vi "Write Averaging time.vi"(8 "error in (no error)":errorcluster, 10 "Time constant":dbl, 11 "RP Lockin in":refnum<class "RP Transceiver.lvclass">) -> (0 "error out":errorcluster, 3 "RP Lockin out":refnum<class "RP Transceiver.lvclass">)   [LabVIEW 2015, in "RP Transceiver.lvclass"]
uses:
  RP Transceiver.lvclass
  RP Transceiver.lvclass/RP Transceiver.ctl
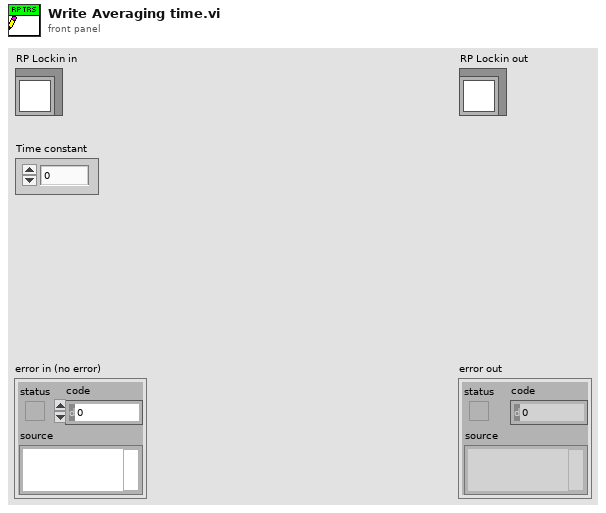
[diagram p1: front panel]
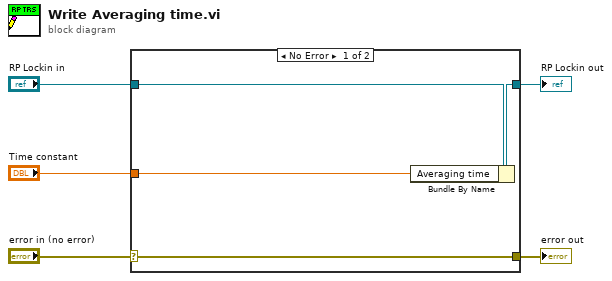
[diagram p0: block diagram]
diagram:
  n1 = case shown="No Error" "error in (no error)" {
    selector: "error in (no error)" -> [w9 w10]
    tunnel: [w9 w10] -> w4
    tunnel: [w7 w11] -> w2
    tunnel: "RP Lockin in" -> [w8 w11]
    tunnel: "Time constant" -> [w6 _]
    frame No Error {
      n2 = Bundle By Name(cluster=w8, "Averaging time"=w6) -> (w7:refnum<class "RP Transceiver.lvclass">)
    }
    frame Error {
    }
  }
  "error out" <- w4
  "RP Lockin out" <- w2
